vi "Kalkulator.vi"() -> ()   [LabVIEW 2023]
panel:
  out "Wynik dzialania":dbl
  in  "STOP":bool
  in  "Dzielenie":bool
  in  "Mnozenie":bool
  in  "Odejmowanie":bool
  in  "Dodawanie":bool
  in  "Num2":dbl
  in  "Num1":dbl
  # "Jaka chcesz przeprowadzic operacje na tych dwoch liczbach?"
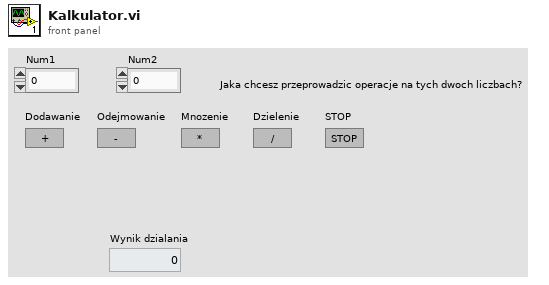
[diagram p1: front panel]
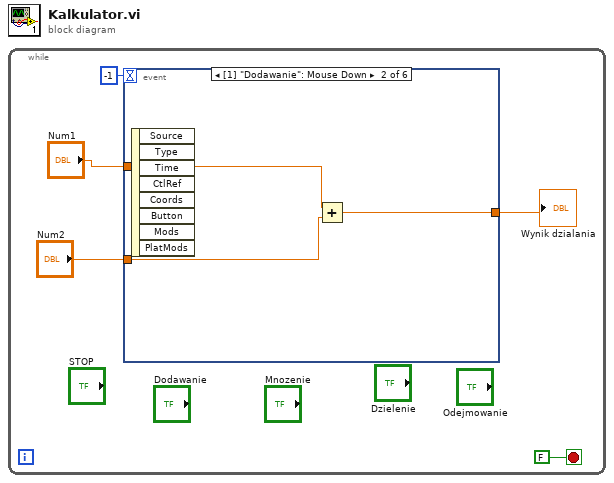
[diagram p0: block diagram]
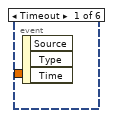
[diagram p2: hidden frame]
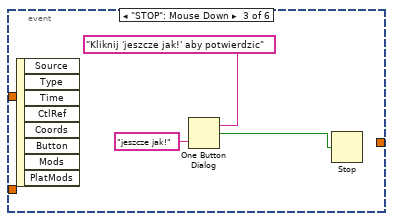
[diagram p3: hidden frame]
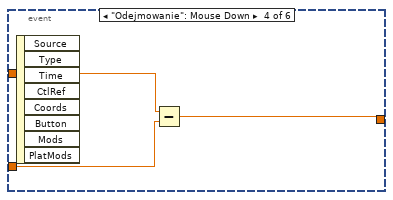
[diagram p4: hidden frame]
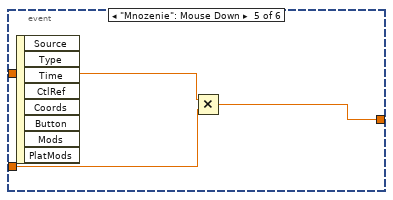
[diagram p5: hidden frame]
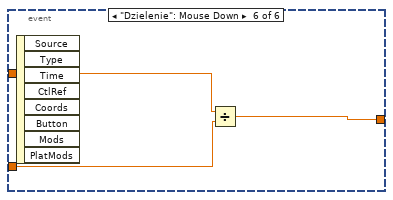
[diagram p6: hidden frame]
diagram:
  n1 = while {
    stop <- FALSE stop-if-true
    n2 = event shown="[1] \"Dodawanie\": Mouse Down" {
      selector: _ -> [_ _ _ _ _ _]
      dyn-events: _ -> [_ _ _ _ _ _]
      timeout: -1 -> [_ _ _ _ _ _]
      tunnel: "Num1" -> [_ w8 _ w14 w17 w20]
      tunnel: "Num2" -> [_ w7 _ w13 w16 w19]
      tunnel: [_ w6 _ w12 w15 w18] -> w1
      event Timeout {
        n3 = event-data() -> ()  [unwired: 1 in, 3 out]
      }
      event "Dodawanie": Mouse Down {
        n4 = event-data() -> ()  [unwired: 1 in, 8 out]
        n5 = Add(x=w8, y=w7) -> (x+y=w6:dbl)
      }
      event "STOP": Mouse Down {
        n6 = event-data() -> ()  [unwired: 1 in, 8 out]
        n7 = One Button Dialog(message="Kliknij 'jeszcze jak!' aby potwierdzic", button name ("OK")="jeszcze jak!") -> (true=w9:bool)
        n8 = Stop(stop? (T)=w9) -> ()
      }
      event "Odejmowanie": Mouse Down {
        n9 = event-data() -> ()  [unwired: 1 in, 8 out]
        n10 = Subtract(x=w14, y=w13) -> (x-y=w12:dbl)
      }
      event "Mnozenie": Mouse Down {
        n11 = event-data() -> ()  [unwired: 1 in, 8 out]
        n12 = Multiply(x=w17, y=w16) -> (x*y=w15:dbl)
      }
      event "Dzielenie": Mouse Down {
        n13 = event-data() -> ()  [unwired: 1 in, 8 out]
        n14 = Divide(x=w20, y=w19) -> (x/y=w18:dbl)
      }
    }
    "Wynik dzialania" <- w1
  }
